vi "Send_Event.vi"(7 "cmd":string, 8 "Error in":errorcluster, 9 "Data":variant, 11 "User Event in":refnum<user-event>) -> (0 "error out":errorcluster, 3 "User Event out":refnum<user-event>)   [LabVIEW 2021]
uses:
  typedef/Queue_Cluster.ctl
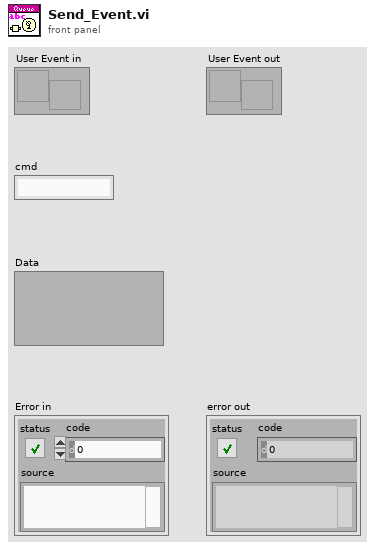
[diagram p1: front panel]
types:
  T1 = typedef "Queue_Cluster.ctl" = cluster{"cmd":string, "Data":variant}
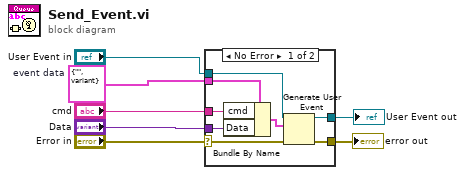
[diagram p0: block diagram]
diagram:
  w5 = T1 {"cmd"="", "Data"=variant}  # event data
  n1 = case shown="No Error" "Error in" {
    selector: "Error in" -> [w10 w16]
    tunnel: "Data" -> [w14 _]
    tunnel: "cmd" -> [w13 _]
    tunnel: w5 -> [w12 _]
    tunnel: "User Event in" -> [w11 w17]
    tunnel: [w9 w16] -> w2
    tunnel: [w8 w17] -> w1
    frame No Error {
      n2 = Bundle By Name(cluster=w12, "cmd"=w13, "Data"=w14) -> (w15:T1)
      n3 = Generate User Event(user event=w11, event data cluster=w15, error in=w10) -> (user event out=w8:refnum<user-event>, error out=w9:errorcluster)  [unwired: 1 in]
    }
    frame Error {
    }
  }
  "error out" <- w2
  "User Event out" <- w1
